vi "Set value by Column.vi"(8 "error in (no error)":errorcluster, 10 "Value Column":refnum<class "Column Interface.lvclass">, 11 "Column in":refnum<class "Column.lvclass">) -> (0 "error out":errorcluster, 3 "Column out":refnum<class "Column.lvclass">)   [LabVIEW 2020, in "Basic Columns.lvlib" / "Column.lvclass"]
uses:
  Column.lvclass
  Column Interface/Column Interface Class/Column Interface.lvclass
  Column.lvclass/Column.ctl
  Database Interfaces/Database Interface Class/Database Interface.lvclass
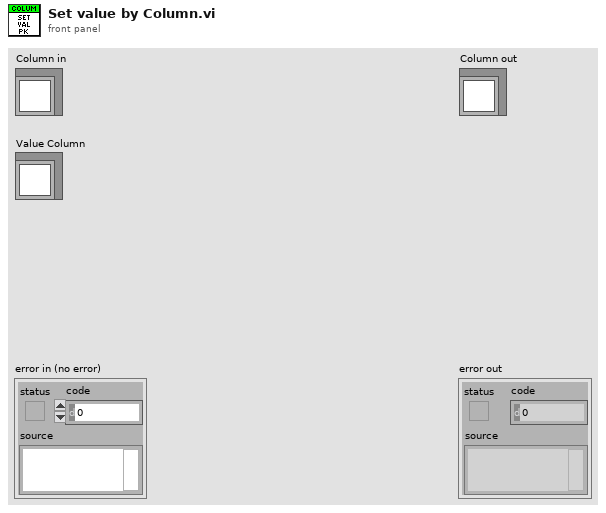
[diagram p1: front panel]
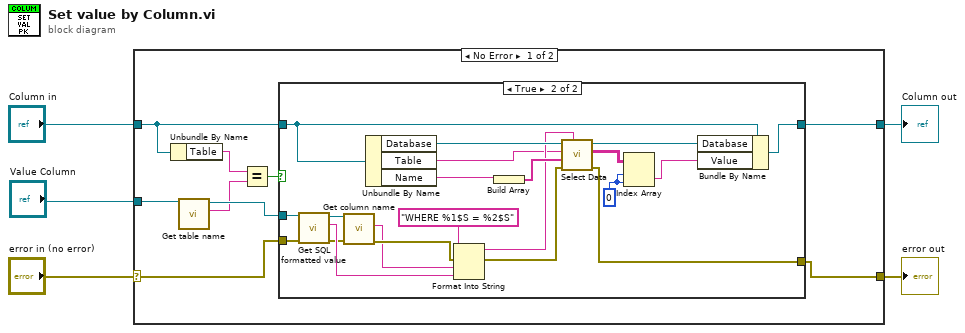
[diagram p0: block diagram]
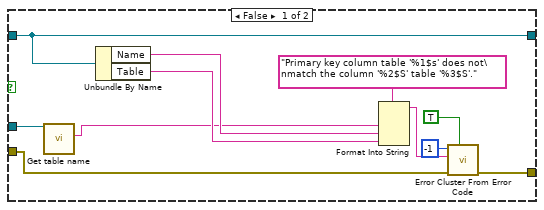
[diagram p2: hidden frame]
diagram:
  n1 = case shown="No Error" "error in (no error)" {
    selector: "error in (no error)" -> [w11 w48]
    tunnel: [w9 w48] -> w4
    tunnel: [w10 w47] -> w2
    tunnel: "Column in" -> [w12 w47]
    tunnel: "Value Column" -> [w8 _]
    frame No Error {
      n2 = Unbundle By Name(w12) -> ("Table"=w14:string)
      n3 = call-dynamic "Get table name.vi"("Column Interface in"=w8) -> ("Table Name"=w6:string, "Column Interface out"=w7:refnum<class "Column Interface.lvclass">)  [unwired: 8 in, 1 out]
      n4 = Equal?(x=w14, y=w6) -> (x = y?=w13:bool)
      n5 = case shown="True" w13 {
        tunnel: w7 -> [w16 w44]
        tunnel: w12 -> [w25 w31]
        tunnel: w11 -> [w17 w37]
        tunnel: [w25 w28] -> w10
        tunnel: [w19 w27] -> w9
        frame False {
          n6 = call-dynamic "Get table name.vi"("Column Interface in"=w16) -> ("Table Name"=w15:string)  [unwired: 8 in, 2 out]
          n7 = Unbundle By Name(w25) -> ("Name"=w23:string, "Table"=w22:string)
          n8 = Format Into String(format string="Primary key column table '%1$s' does not\nmatch the column '%2$S' table '%3$S'.", w15, w23, w22) -> (resulting string=w21:string)  [unwired: 2 in, 1 out]
          n9 = call <vilib>:"Error Cluster From Error Code.vi"("show call chain? (False)"=TRUE, "error in (no error)"=w17, "error message (\"\")"=w21, "error code (0)"=-1) -> ("error out"=w19:errorcluster)  [unwired: 5 in]
        }
        frame True {
          w32 = 0 ("index (row)")
          n10 = call-dynamic "Get SQL formatted value.vi"("error in (no error)"=w37, "Column Interface in"=w44) -> ("error out"=w36:errorcluster, "Formatted Value"=w45:string, "Column Interface out"=w43:refnum<class "Column Interface.lvclass">)  [unwired: 7 in]
          n11 = call-dynamic "Get column name.vi"("error in (no error)"=w36, "Column Interface in"=w43) -> ("error out"=w35:errorcluster, "Name"=w26:string)  [unwired: 7 in, 1 out]
          n12 = Unbundle By Name(w31) -> ("Database"=w40:refnum<class "Database Interface.lvclass">, "Table"=w38:string, "Name"=w42:string)
          n13 = Format Into String(initial string="WHERE %1$S = %2$S", error in=w35, w26, w45) -> (resulting string=w39:string, error out=w34:errorcluster)  [unwired: 1 in]
          n14 = Build Array(w42) -> (w41:string[])
          n15 = call-dynamic "Select Data.vi"("WHERE Statement"=w39, "error in (no error)"=w34, "Columns"=w41, "Table"=w38, "Database Interface in"=w40) -> ("error out"=w27:errorcluster, "Data"=w33:string[][], "Database Interface out"=w30:refnum<class "Database Interface.lvclass">)  [unwired: 4 in]
          n16 = Index Array(array=w33, index (row)=w32, index (col)=w32) -> (element=w29:string)
          n17 = Bundle By Name(cluster=w31, "Database"=w30, "Value"=w29) -> (w28:refnum<class "Column.lvclass">)
        }
      }
    }
    frame Error {
    }
  }
  "error out" <- w4
  "Column out" <- w2
